vi "LVClass_CorrectionDataManager Load InteractrionMatrix.vi"(0 "CorrectionDataManager in":refnum<class "CorrectionDataManager.lvclass">, 7 "Interaction Matrix file path":path, 11 "error in (no error)":errorcluster) -> (4 "CorrectionDataManager out":refnum<class "CorrectionDataManager.lvclass">, 15 "error out":errorcluster)   [LabVIEW 2020, in "CorrectionDataManager.lvclass"]
doc: "Load data extracted from a CorrDataManager backup file into current\nCorrDataManager object.\n\n<B>corrdata_managerIn</B> : CorrDataManager object.\n<B>corrdata_managerOut</B> : CorrDataManager object.\n<B>backup_file_path</B> : Absolute path to CorrDataManager backup file."
uses:
  CorrectionDataManager.lvclass
  CorrectionDataManager.lvclass/CorrectionDataManager.ctl
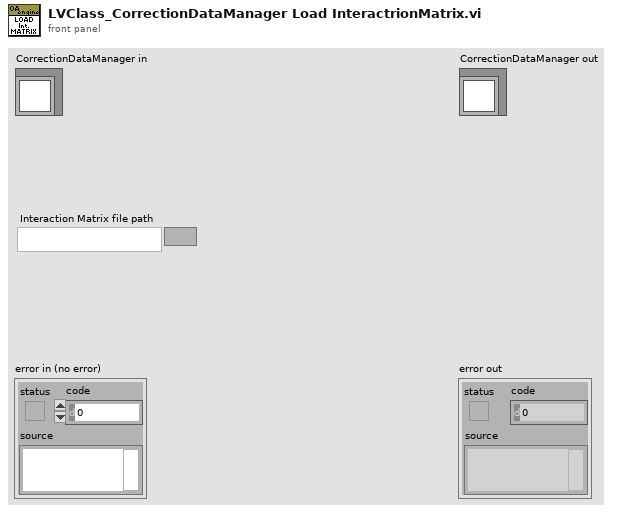
[diagram p1: front panel]
types:
  T1 = typedef "ClassID.ctl" = i64
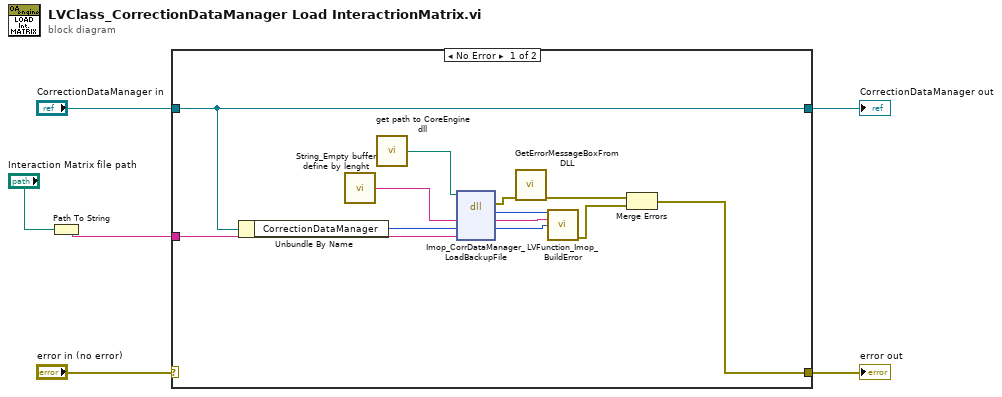
[diagram p0: block diagram]
diagram:
  n1 = Path To String(path="Interaction Matrix file path") -> (string=w1:string)
  n2 = case shown="No Error" "error in (no error)" {
    selector: "error in (no error)" -> [_ w20]
    tunnel: [w10 w20] -> w3
    tunnel: [w11 w19] -> w6
    tunnel: "CorrectionDataManager in" -> [w11 w19]
    tunnel: w1 -> [w8 _]
    frame No Error {
      n3 = Unbundle By Name(w11) -> ("CorrectionDataManager"=w9:T1)
      n4 = call "String_Empty buffer define by lenght.vi"() -> ("Empty buffer"=w16:string)  [unwired: 1 in]
      n5 = call "get path to CoreEngine dll.vi"() -> ("path to wavekit library"=w15:path)  [unwired: 14 in, 1 out]
      n6 = dll-call lib="D:/soft/HASO_v3/SVN_trunk/ImOpCoreEngine4_LV2011/DLLs/c_interface_vc100.dll" fn="Imop_CorrDataManager_LoadBackupFile"(path in=w15, "message"=w16, "WavefrontCorrection"=w9, "IM filename"=w8) -> (error out=w14:errorcluster, "return type"=w18:i32, "message"=w17:string, "WavefrontCorrection"=w7:i64)  [unwired: 3 in, 1 out]
      n7 = call "GetErrorMessageBoxFromDLL.vi"("error IN"=w14) -> ("error OUT"=w13:errorcluster)  [unwired: 10 in]
      n8 = call "LVFunction_Imop_BuildError.vi"("code"=w18, "String to Prepend to source (\"\")"=w17, "Adresse"=w7) -> ("error out"=w12:errorcluster)  [unwired: 12 in]
      n9 = Merge Errors(w13, w12) -> (w10:errorcluster)
    }
    frame Error {
    }
  }
  "error out" <- w3
  "CorrectionDataManager out" <- w6
